vi "Calculate Average Sector Background.vi"(8 "error in (no error)":errorcluster, 9 "Image":T1, 10 "Right Sector Parameters":T3, 11 "Left Sector Parameters":T3) -> (0 "error out":errorcluster, 2 "Canceled?":bool, 3 "[Avg BG]":dbl[](array[numeric]))   [LabVIEW 2013]
uses:
  FPGA/Sector/Accumulate/Sector Parameter Cluster.ctl
  FPGA/Sector/Accumulate/Accumulated Sector Cluster.ctl
  <vilib>/vision/Image Controls.llb/IMAQ Image.ctl
panel:
  out "Accumulated BG":T2[](array[typedef])
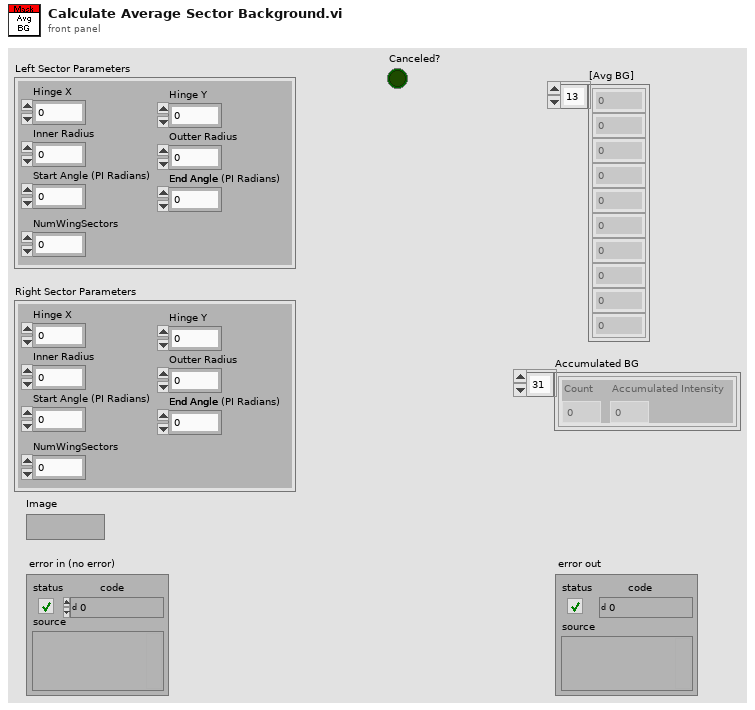
[diagram p1: front panel]
types:
  T1 = typedef "IMAQ Image.ctl" = refnum<image>
  T2 = typedef "Accumulated Sector Cluster.ctl" = cluster{"Accumulated Intensity":u32, "Count":u16}
  T3 = typedef "Sector Parameter Cluster.ctl" = cluster{"Start Angle":fxp<+/-,17,2>, "End Angle":fxp<+/-,17,2>, "Inner Radius":u16, "Outter Radius":u16, "Hinge X":u16, "Hinge Y":u16, "NumWingSectors":u8}
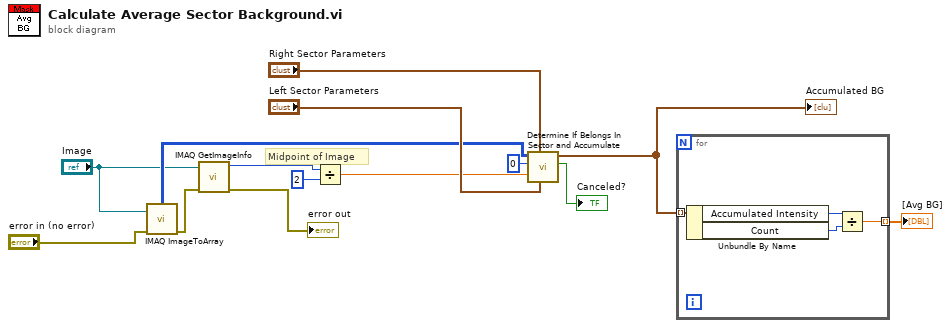
[diagram p0: block diagram]
diagram:
  # "Midpoint of Image"
  n1 = call "IMAQ ImageToArray"("error in (no error)"="error in (no error)", "Image"="Image") -> ("error out"=w6:errorcluster, "Image Pixels (U8)"=w4:u8[][])  [unwired: 2 in, 3 out]
  n2 = call "IMAQ GetImageInfo"("error in (no error)"=w6, "Image"="Image") -> ("error out"=→"error out":errorcluster, "X Resolution"=w14:i32)  [unwired: 2 in, 6 out]
  n3 = Divide(x=w14, y=2) -> (x/y=w9:dbl)
  n4 = call "Determine If Belongs In Sector and Accumulate.vi"("Left Sector Parameters"="Left Sector Parameters", "Right Sector Parameters"="Right Sector Parameters", "Midpoint of Image"=w9, "Starting Y Location"=0, "Image Data"=w4) -> ("Canceled?"=→"Canceled?":bool, "[Accumulated Sectors]"=w3:T2[])  [unwired: 4 in, 1 out]
  "Accumulated BG" <- w3
  n5 = for {
    tunnel: w3 -> [w18] mode=indexing
    tunnel: [w15] -> w8 mode=indexing
    n6 = Unbundle By Name(w18) -> ("Accumulated Intensity"=w17:u32, "Count"=w16:u16)
    n7 = Divide(x=w17, y=w16) -> (x/y=w15:dbl)
  }
  "[Avg BG]" <- w8
